vi "apply autoconfigure sensor config.vi"(10 "ds_handle":u32, 11 "context":u32) -> (1 "function return":i32, 2 "ds_handle out":u32, 3 "context out":u32)   [LabVIEW 2019, in "apdm.lvlib"]
doc: "APDM_EXPORT int apdm_apply_autoconfigure_sensor_config(apdm_ctx_t context, apdm_device_handle_t ds_handle);"
uses:
  apdm.lvlib
  Lee Lab/CP FES Walking 2018/Code/Working/LabVIEW/apdm.dll
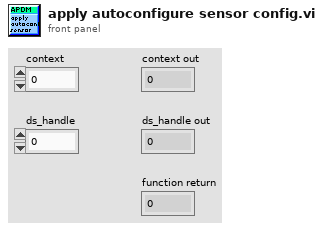
[diagram p1: front panel]
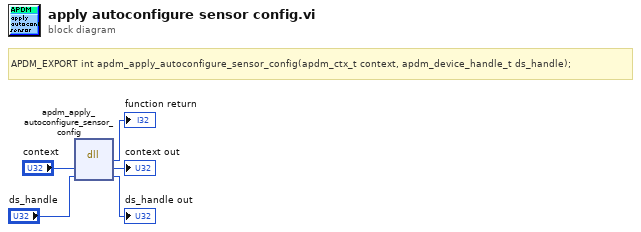
[diagram p0: block diagram]
diagram:
  # "APDM_EXPORT int apdm_apply_autoconfigure_sensor_config(apdm_ctx_t context, apdm_device_handle_t ds_handle);"
  n1 = dll-call lib="C:/Users/jfalesi/Dropbox/Lee Lab/CP FES Walking 2018/Code/Working/LabVIEW/apdm.*" fn="apdm_apply_autoconfigure_sensor_config"("context"="context", "ds_handle"="ds_handle") -> (→"function return":i32, "context"=→"context out":u32, "ds_handle"=→"ds_handle out":u32)  [unwired: 3 in, 2 out]
